vi "sat_H2O_vap_press_2024.vi"(2 "Saturation below 273.16 K":i32(listbox), 3 "Temperature [K]":dbl=373.15 format="%.5g") -> (0 "saturated water vapor pressure [atm]":dbl=1.0009281197694644 format="%.5g", 1 "saturated water vapor pressure [Pa]":dbl=101419.04173564097 format="%.2f")   [LabVIEW 2016]
uses:
  <vilib>/gmath/NI_Gmath.lvlib
panel:
  out "saturated water vapor pressure [kPa]":dbl=101.41904173564097 format="%_6g"
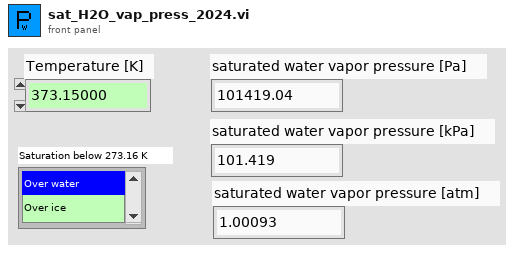
[diagram p1: front panel]
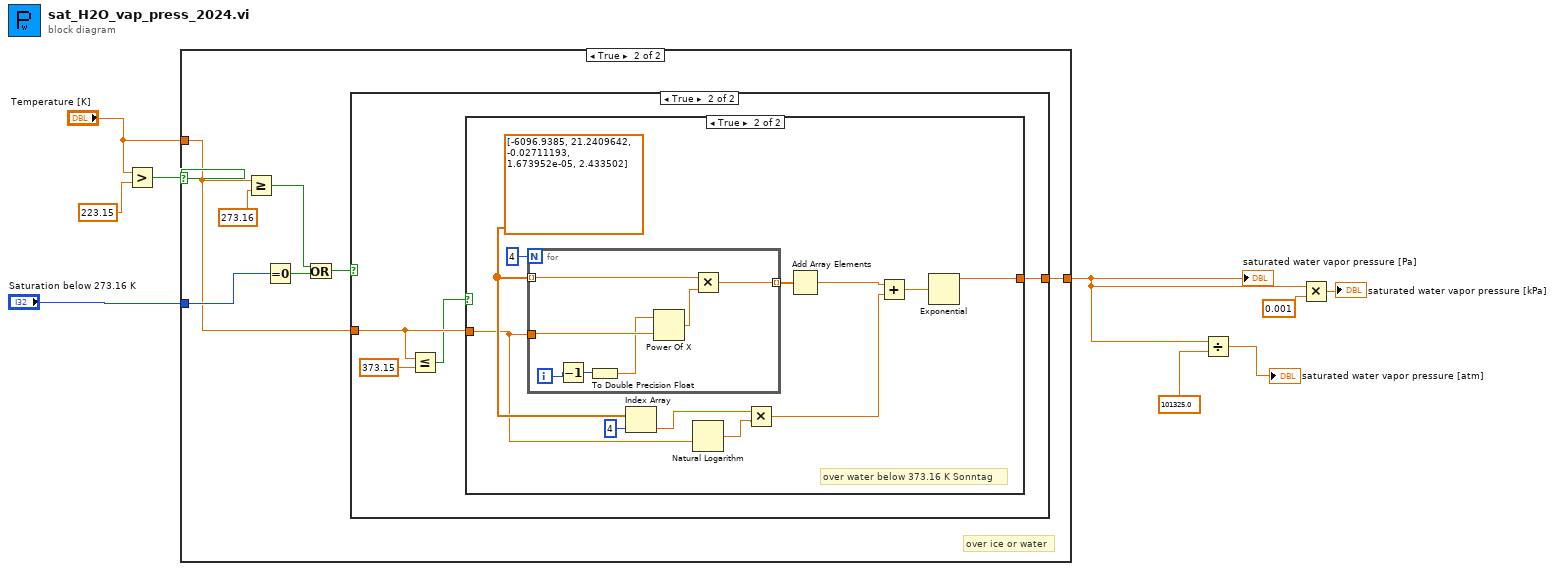
[diagram p0: block diagram]
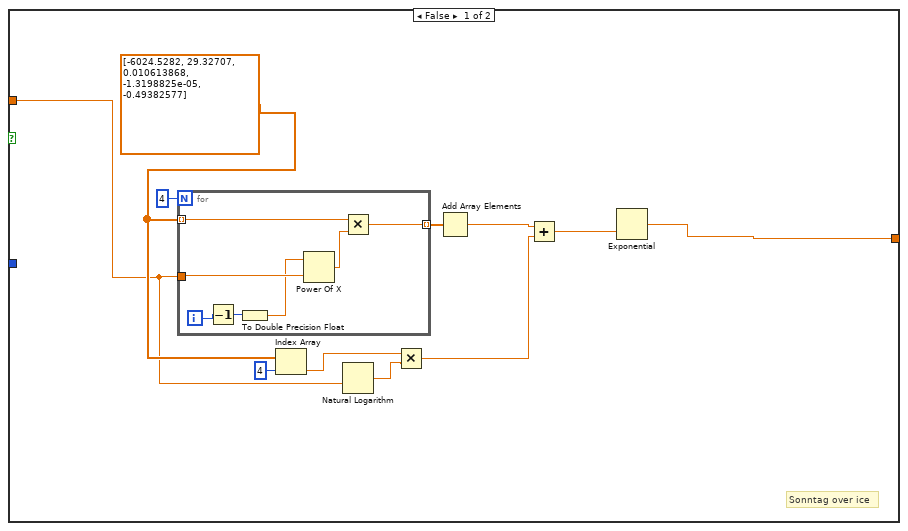
[diagram p2: hidden frame]
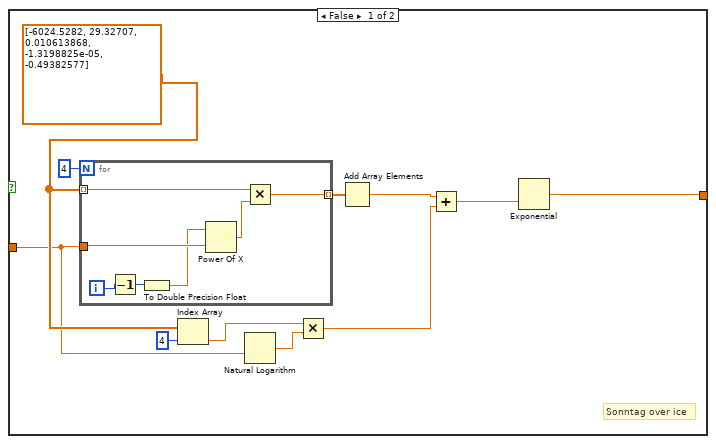
[diagram p3: hidden frame]
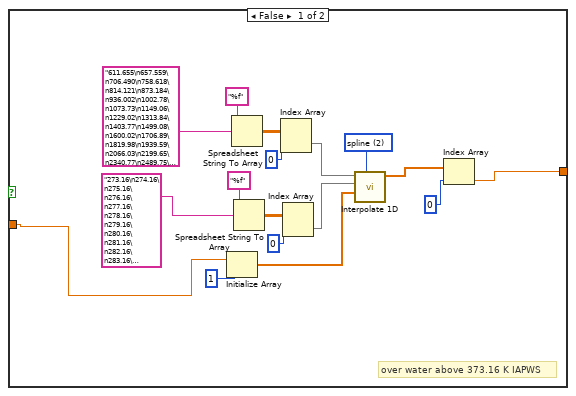
[diagram p4: hidden frame]
diagram:
  n1 = Greater?(x="Temperature [K]", y=223.15) -> (0:w6:bool)
  n2 = case shown="True" w6 {
    tunnel: "Temperature [K]" -> [w11 w28]
    tunnel: "Saturation below 273.16 K" -> [_ w32]
    tunnel: [w10 w29] -> w4
    frame False {
      w13 = dbl[] [-6024.5282, 29.32707, 0.010613868, -1.3198825e-05, -0.49382577]
      # "Sonntag over ice"
      n3 = for {
        N: 4 -> [_]
        tunnel: w13 -> [w27] mode=indexing
        tunnel: w11 -> [w26]
        tunnel: [w21] -> w19 mode=indexing
        i -> [w25]
        n4 = Decrement(x=w25) -> (x-1=w24:i32)
        n5 = To Double Precision Float(number=w24) -> (double precision float=w23:dbl)
        n6 = Power Of X(1:w26, 2:w23) -> (0:w22:dbl)
        n7 = Multiply(x=w27, y=w22) -> (x*y=w21:dbl)
      }
      n8 = Index Array(array=w13, index=4) -> (element=w16:dbl)
      n9 = Natural Logarithm(1:w11) -> (0:w17:dbl)
      n10 = Multiply(x=w16, y=w17) -> (x*y=w14:dbl)
      n11 = Add Array Elements(numeric array=w19) -> (sum=w15:dbl)
      n12 = Add(x=w15, y=w14) -> (x+y=w12:dbl)
      n13 = Exponential(1:w12) -> (0:w10:dbl)
    }
    frame True {
      # "over ice or water"
      n14 = Greater Or Equal?(x=w28, y=273.16) -> (x >= y?=w33:bool)
      n15 = Equal To 0?(x=w32) -> (x = 0?=w31:bool)
      n16 = Or(x=w33, y=w31) -> (x .or. y?=w30:bool)
      n17 = case shown="True" w30 {
        tunnel: [w35 w56] -> w29
        tunnel: w28 -> [w37 w54]
        frame False {
          w38 = dbl[] [-6024.5282, 29.32707, 0.010613868, -1.3198825e-05, -0.49382577]
          # "Sonntag over ice"
          n18 = for {
            N: 4 -> [_]
            tunnel: w38 -> [w52] mode=indexing
            tunnel: w37 -> [w51]
            tunnel: [w46] -> w44 mode=indexing
            i -> [w50]
            n19 = Decrement(x=w50) -> (x-1=w49:i32)
            n20 = To Double Precision Float(number=w49) -> (double precision float=w48:dbl)
            n21 = Power Of X(1:w51, 2:w48) -> (0:w47:dbl)
            n22 = Multiply(x=w52, y=w47) -> (x*y=w46:dbl)
          }
          n23 = Index Array(array=w38, index=4) -> (element=w41:dbl)
          n24 = Natural Logarithm(1:w37) -> (0:w42:dbl)
          n25 = Multiply(x=w41, y=w42) -> (x*y=w39:dbl)
          n26 = Add Array Elements(numeric array=w44) -> (sum=w40:dbl)
          n27 = Add(x=w40, y=w39) -> (x+y=w36:dbl)
          n28 = Exponential(1:w36) -> (0:w35:dbl)
        }
        frame True {
          n29 = Less Or Equal?(x=w54, y=373.15) -> (x <= y?=w53:bool)
          n30 = case shown="True" w53 {
            tunnel: [w57 w84] -> w56
            tunnel: w54 -> [w58 w79]
            frame False {
              w59 = 2 items=["nearest", "linear", "spline", "cubic Hermite", "Lagrange"] ("method")
              # "over water above 373.16 K IAPWS"
              n31 = Initialize Array(w58, 1 ("dimension size")) -> (w72:dbl[])
              n32 = Spreadsheet String To Array(format string="%f", spreadsheet string="611.655\n657.559\n706.490\n758.618\n814.121\n873.184\n936.002\n1002.78\n1073.73\n1149.06\n1229.02\n1313.84\n1403.77\n1499.08\n1600.02\n1706.89\n1819.98\n1939.59\n2066.03\n2199.65\n2340.77\n2489.75\n2646.96\n2812.77\n2987.59\n3171.82\n3365.88\n3570.21\n3785.26\n4011.50\n4249.41\n4499.49\n4762.27\n5038.26\n5328.03\n5632.13\n5951.16\n6285.72\n6636.42\n7003.92\n7388.88\n7791.96\n8213.88\n8655.35\n9117.11\n9599.93\n10104.6\n10631.9\n11182.7\n11757.8\n12358.1\n12984.5\n13637.9\n14319.2\n15029.5\n15769.7\n16540.8\n17343.8\n18179.9\n19050.2\n19955.7\n20897.5\n21877.0\n22895.2\n23953.4\n25052.8\n26194.8\n27380.5\n28611.5\n29889.0\n31214.4\n32589.2\n34014.8\n35492.7\n37024.5\n38611.5\n40255.6\n41958.1\n43720.9\n45545.5\n47433.7\n49387.1\n51407.6\n53497.0\n55657.1\n57889.7\n60196.7\n62580.1\n65041.9\n67584.0\n70208.4\n72917.3\n75712.7\n78596.8\n81571.7\n84639.6\n87802.8\n91063.5\n94424.1\n97886.9\n101454.\n105128.\n108912.\n112808.\n116818.\n120945.\n125192.\n129560.\n134054.\n138675.\n143427.\n148312.\n153332.\n158491.\n163792.\n169238.\n174830.\n180574.\n186471.\n192524.\n198737.\n205113.\n211655.\n218367.\n225250.\n232310.\n239548.\n246969.\n254576.\n262372.\n270361.\n278546.\n286931.\n295519.\n304315.\n313321.\n322541.\n331979.\n341640.\n351526.\n361641.\n371990.\n382577.\n393404.\n404477.\n415799.\n427375.\n439207.\n451302.\n463662.\n476292.\n489197.\n502379.\n515845.\n529598.\n543642.\n557982.\n572623.\n587568.\n602823.\n618392.\n634279.\n650490.\n667029.\n683900.\n701108.\n718659.\n736556.\n754805.\n773411.\n792378.\n811712.\n831418.\n851499.\n871963.\n892813.\n914054.\n935693.\n957733.\n980181.\n1003040.\n1026320.\n1050020.\n1074150.\n1098710.\n1123720.\n1149160.\n1175060.\n1201420.\n1228230.\n1255510.\n1283270.\n1311500.\n1340210.\n1369420.\n1399120.\n1429320.\n1460030.\n1491250.\n1522990.\n1555250.\n1588050.\n1621380.\n1655250.\n1689670.\n1724650.\n1760180.\n1796290.\n1832960.\n1870220.\n1908060.\n1946490.\n1985520.\n2025150.\n2065390.\n2106250.\n2147740.\n2189850.\n2232600.\n2275990.\n2320030.\n2364730.\n2410080.\n2456110.\n2502820.\n2550200.\n2598280.\n2647050.\n2696520.\n2746700.\n2797600.\n2849220.\n2901570.\n2954660.\n3008500.\n3063080.\n3118420.\n3174530.\n3231410.\n3289070.\n3347510.\n3406750.\n3466790.\n3527640.\n3589310.\n3651800.\n3715120.\n3779270.\n3844280.\n3910130.\n3976850.\n4044430.\n4112890.\n4182230.\n4252470.\n4323600.\n4395640.\n4468590.\n4542470.\n4617280.\n4693020.\n4769710.\n4847360.\n4925970.\n5005540.\n5086100.\n5167640.\n5250180.\n5333720.\n5418280.\n5503850.\n5590450.\n5678090.\n5766770.\n5856510.\n5947310.\n6039180.\n6132130.\n6226170.\n6321310.\n6417550.\n6514910.\n6613400.\n6713010.\n6813770.\n6915690.\n7018760.\n7123010.\n7228430.\n7335050.\n7442860.\n7551890.\n7662130.\n7773600.\n7886300.\n8000260.\n8115470.\n8231960.\n8349720.\n8468770.\n8589110.\n8710770.\n8833750.\n8958060.\n9083710.\n9210710.\n9339080.\n9468820.\n9599940.\n9732470.\n9866400.\n10001700.\n10138500.\n10276800.\n10416400.\n10557600.\n10700200.\n10844300.\n10990000.\n11137100.\n11285800.\n11436000.\n11587800.\n11741100.\n11896100.\n12052600.\n12210700.\n12370500.\n12531900.\n12695000.\n12859700.\n13026100.\n13194300.\n13364100.\n13535700.\n13709000.\n13884100.\n14061000.\n14239700.\n14420200.\n14602500.\n14786700.\n14972800.\n15160800.\n15350700.\n15542500.\n15736300.\n15932000.\n16129800.\n16329600.\n16531400.\n16735400.\n16941400.\n17149500.\n17359800.\n17572300.\n17786900.\n18003800.\n18223000.\n18444500.\n18668300.\n18894400.\n19123000.\n19354000.\n19587600.\n19823700.\n20062500.\n20304000.\n20548400.\n20795700.\n21046100.\n21299700.\n21556500.\n21816800.\n") -> (array=w65:dbl[][])  [unwired: 2 in]
              n33 = Spreadsheet String To Array(format string="%f", spreadsheet string="273.16\n274.16\n275.16\n276.16\n277.16\n278.16\n279.16\n280.16\n281.16\n282.16\n283.16\n284.16\n285.16\n286.16\n287.16\n288.16\n289.16\n290.16\n291.16\n292.16\n293.16\n294.16\n295.16\n296.16\n297.16\n298.16\n299.16\n300.16\n301.16\n302.16\n303.16\n304.16\n305.16\n306.16\n307.16\n308.16\n309.16\n310.16\n311.16\n312.16\n313.16\n314.16\n315.16\n316.16\n317.16\n318.16\n319.16\n320.16\n321.16\n322.16\n323.16\n324.16\n325.16\n326.16\n327.16\n328.16\n329.16\n330.16\n331.16\n332.16\n333.16\n334.16\n335.16\n336.16\n337.16\n338.16\n339.16\n340.16\n341.16\n342.16\n343.16\n344.16\n345.16\n346.16\n347.16\n348.16\n349.16\n350.16\n351.16\n352.16\n353.16\n354.16\n355.16\n356.16\n357.16\n358.16\n359.16\n360.16\n361.16\n362.16\n363.16\n364.16\n365.16\n366.16\n367.16\n368.16\n369.16\n370.16\n371.16\n372.16\n373.16\n374.16\n375.16\n376.16\n377.16\n378.16\n379.16\n380.16\n381.16\n382.16\n383.16\n384.16\n385.16\n386.16\n387.16\n388.16\n389.16\n390.16\n391.16\n392.16\n393.16\n394.16\n395.16\n396.16\n397.16\n398.16\n399.16\n400.16\n401.16\n402.16\n403.16\n404.16\n405.16\n406.16\n407.16\n408.16\n409.16\n410.16\n411.16\n412.16\n413.16\n414.16\n415.16\n416.16\n417.16\n418.16\n419.16\n420.16\n421.16\n422.16\n423.16\n424.16\n425.16\n426.16\n427.16\n428.16\n429.16\n430.16\n431.16\n432.16\n433.16\n434.16\n435.16\n436.16\n437.16\n438.16\n439.16\n440.16\n441.16\n442.16\n443.16\n444.16\n445.16\n446.16\n447.16\n448.16\n449.16\n450.16\n451.16\n452.16\n453.16\n454.16\n455.16\n456.16\n457.16\n458.16\n459.16\n460.16\n461.16\n462.16\n463.16\n464.16\n465.16\n466.16\n467.16\n468.16\n469.16\n470.16\n471.16\n472.16\n473.16\n474.16\n475.16\n476.16\n477.16\n478.16\n479.16\n480.16\n481.16\n482.16\n483.16\n484.16\n485.16\n486.16\n487.16\n488.16\n489.16\n490.16\n491.16\n492.16\n493.16\n494.16\n495.16\n496.16\n497.16\n498.16\n499.16\n500.16\n501.16\n502.16\n503.16\n504.16\n505.16\n506.16\n507.16\n508.16\n509.16\n510.16\n511.16\n512.16\n513.16\n514.16\n515.16\n516.16\n517.16\n518.16\n519.16\n520.16\n521.16\n522.16\n523.16\n524.16\n525.16\n526.16\n527.16\n528.16\n529.16\n530.16\n531.16\n532.16\n533.16\n534.16\n535.16\n536.16\n537.16\n538.16\n539.16\n540.16\n541.16\n542.16\n543.16\n544.16\n545.16\n546.16\n547.16\n548.16\n549.16\n550.16\n551.16\n552.16\n553.16\n554.16\n555.16\n556.16\n557.16\n558.16\n559.16\n560.16\n561.16\n562.16\n563.16\n564.16\n565.16\n566.16\n567.16\n568.16\n569.16\n570.16\n571.16\n572.16\n573.16\n574.16\n575.16\n576.16\n577.16\n578.16\n579.16\n580.16\n581.16\n582.16\n583.16\n584.16\n585.16\n586.16\n587.16\n588.16\n589.16\n590.16\n591.16\n592.16\n593.16\n594.16\n595.16\n596.16\n597.16\n598.16\n599.16\n600.16\n601.16\n602.16\n603.16\n604.16\n605.16\n606.16\n607.16\n608.16\n609.16\n610.16\n611.16\n612.16\n613.16\n614.16\n615.16\n616.16\n617.16\n618.16\n619.16\n620.16\n621.16\n622.16\n623.16\n624.16\n625.16\n626.16\n627.16\n628.16\n629.16\n630.16\n631.16\n632.16\n633.16\n634.16\n635.16\n636.16\n637.16\n638.16\n639.16\n640.16\n641.16\n642.16\n643.16\n644.16\n645.16\n646.16") -> (array=w68:dbl[][])  [unwired: 2 in]
              n34 = Index Array(array=w65, index (col)=0 ("disabled index (col)")) -> (element=w62:dbl[])  [unwired: 1 in]
              n35 = Index Array(array=w68, index (col)=0 ("disabled index (col)")) -> (element=w63:dbl[])  [unwired: 1 in]
              n36 = call <vilib>:"Interpolate 1D.vi"("method"=w59, "xi"=w72, "X"=w63, "Y"=w62) -> ("yi"=w71:dbl[])  [unwired: 5 in, 2 out]
              n37 = Index Array(array=w71, index=0) -> (element=w57:dbl)
            }
            frame True {
              w81 = dbl[] [-6096.9385, 21.2409642, -0.02711193, 1.673952e-05, 2.433502]
              # "over water below 373.16 K Sonntag"
              n38 = for {
                N: 4 -> [_]
                tunnel: w81 -> [w91] mode=indexing
                tunnel: w79 -> [w90]
                tunnel: [w85] -> w82 mode=indexing
                i -> [w89]
                n39 = Decrement(x=w89) -> (x-1=w88:i32)
                n40 = To Double Precision Float(number=w88) -> (double precision float=w87:dbl)
                n41 = Power Of X(1:w90, 2:w87) -> (0:w86:dbl)
                n42 = Multiply(x=w91, y=w86) -> (x*y=w85:dbl)
              }
              n43 = Index Array(array=w81, index=4) -> (element=w77:dbl)
              n44 = Natural Logarithm(1:w79) -> (0:w78:dbl)
              n45 = Multiply(x=w77, y=w78) -> (x*y=w75:dbl)
              n46 = Add Array Elements(numeric array=w82) -> (sum=w76:dbl)
              n47 = Add(x=w76, y=w75) -> (x+y=w74:dbl)
              n48 = Exponential(1:w74) -> (0:w84:dbl)
            }
          }
        }
      }
    }
  }
  "saturated water vapor pressure [Pa]" <- w4
  n49 = Divide(x=w4, y=101325.0 ("x")) -> (x/y=→"saturated water vapor pressure [atm]":dbl)
  n50 = Multiply(x=w4, y=0.001) -> (x*y=→"saturated water vapor pressure [kPa]":dbl)
